vi "Data Set Units.vi"(8 "error in (no error)":errorcluster, 10 "Units":refnum<data-value>, 11 "Data DVR in":refnum<data-value>) -> (0 "error out":errorcluster, 3 "Data DVR out":refnum<data-value>)   [LabVIEW 2012, in "MDSplus.lvlib"]
doc: "Set the Units field for this Data instance."
uses:
  <vilib>/MDSplus/Library/MDSplus.lvlib
  <vilib>/MDSplus/Classes/Data_Class/Data.lvclass
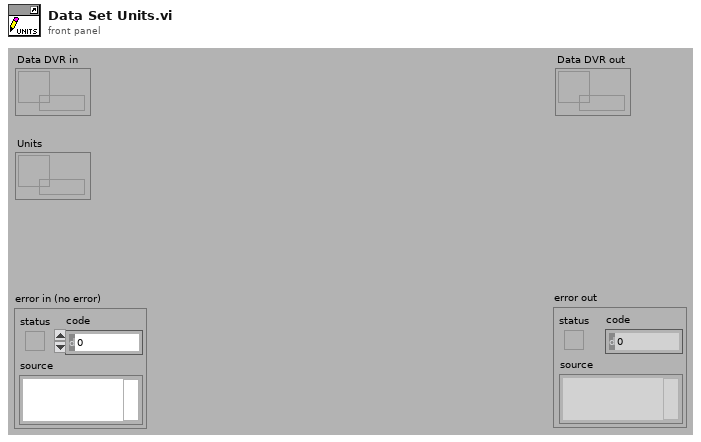
[diagram p1: front panel]
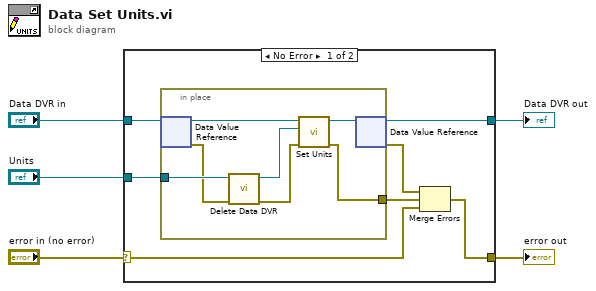
[diagram p0: block diagram]
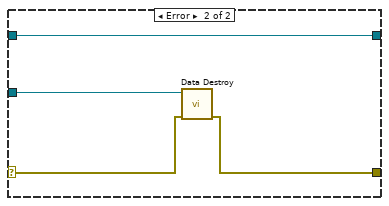
[diagram p2: hidden frame]
diagram:
  n1 = case shown="No Error" "error in (no error)" {
    selector: "error in (no error)" -> [w11 w21]
    tunnel: "Data DVR in" -> [w12 w23]
    tunnel: [w8 w20] -> w5
    tunnel: [w9 w23] -> w2
    tunnel: "Units" -> [w6 w22]
    frame No Error {
      n2 = in-place {
        in-place-border: [w13] -> w7
        in-place-border: w6 -> [w17]
        n3 = in-place-dvr #1(w12) -> (w19:refnum<class "Data.lvclass">, w16:errorcluster)
        n4 = call <vilib>:"Delete Data DVR.vi"("error in (no error)"=w16, "Data DVR in"=w17) -> ("error out"=w15:errorcluster, "Data out"=w14:refnum<class "Data.lvclass">)  [unwired: 8 in]
        n5 = call-dynamic "Set Units.vi"("error in (no error)"=w15, "Units"=w14, "Data in"=w19) -> ("error out"=w13:errorcluster, "Data out"=w18:refnum<class "Data.lvclass">)  [unwired: 7 in]
        n6 = in-place-dvr #1(w18) -> (w9:refnum<data-value>, w10:errorcluster)
      }
      n7 = Merge Errors(w10, w7, w11) -> (w8:errorcluster)
    }
    frame Error {
      n8 = call <vilib>:"Data Destroy.vi"("error in (no error)"=w21, "Data DVR in"=w22) -> ("error out"=w20:errorcluster)  [unwired: 9 in]
    }
  }
  "error out" <- w5
  "Data DVR out" <- w2
